vi "_readLabel_fromDatabase_wmg.vi"(0 "input_str_label":string="11S90Y9428Y050YW6154M1", 1 "SN keep":bool, 2 "date":timestamp, 3 "input_array_labelConfig":string[](array[string])=["年月日", "16", "16", "17", "17", "", "", "18", "18", "19", "21", "Y050YW(YMD)(S3)"]) -> (4 "show_str_yywwSd":string, 5 "show_str_yydddxxxx":string, 6 "show_int_Xn":i32, 7 "show_date":timestamp format="%<%X\n%x>T", 8 "show_str_snObeyFormat":string="LR5AN0021")   [LabVIEW 2011]
panel:
  in  "midVar_date_2":timestamp
  in  "midVar_date_1":timestamp
  # "周日是一周的第0天"
  # "1904050897/Z00A2R1543S500016\n0       5       10         17     22\nL99SF014-SD-H"
  # "8SSC10G59338L1DG5AN0004\nL01HE006-SD-R"
  # "1904050897/Z00A2R1543S500016\n0       5       10         17     22\nL99SF014-SD-H\n\n1543S5经本程序计算得到2015/10/23 296"
  # "这个输出接口估计用不到了"
  # "17 18"
  # "数组元素索引\n0  description\n1  yearStart\n2  yearEnd\n3  monthStart\n4  monthEnd\n5  weekStart\n6  weekEnd\n7  DayStart\n8  DayEnd\n9  snStart\n10 snEnd\n11  snFormat\n12  cableType\n13  preStaData\n14  significant\n15  noRetest"
  # "0  description"
  # "1  yearStart"
  # "8SSC10G59338L1DG5AN0004\n\nL01HE006-SD-R\n5AN经本程序计算得到2015/10/22 295\n\n8SSC10G59338L1DG5110004\nL01HE006-SD-R\n5AN经本程序计算得到2015/1/1 1"
  # "2  yearEnd"
  # "3  monthStart"
  # "4  monthEnd"
  # "5  weekStart"
  # "6  weekEnd"
  # "7  DayStart"
  # "8  DayEnd"
  # "9  snStart"
  # "10 snEnd"
  # "11  snFormat"
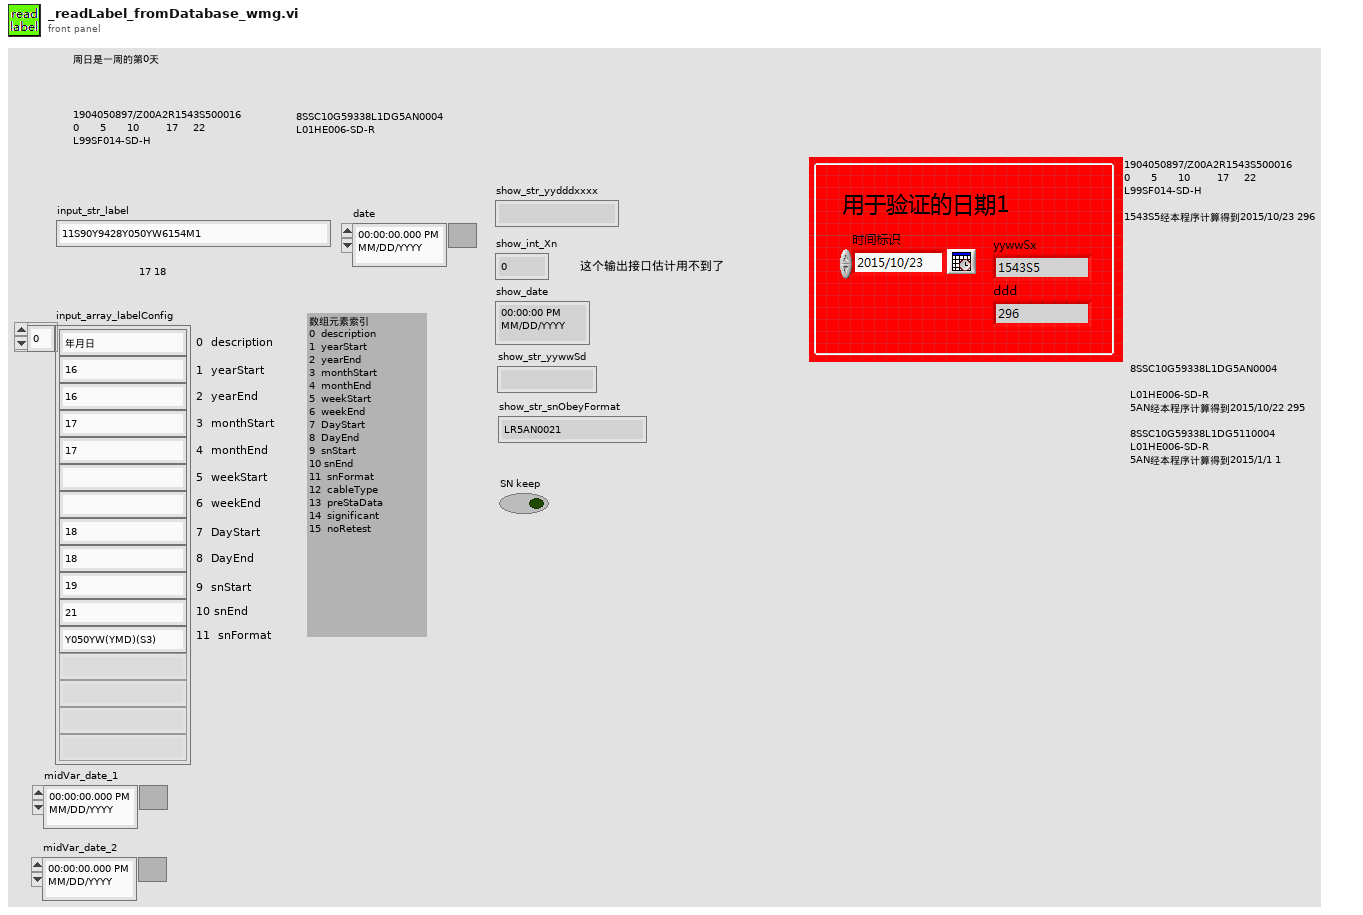
[diagram p1: front panel]
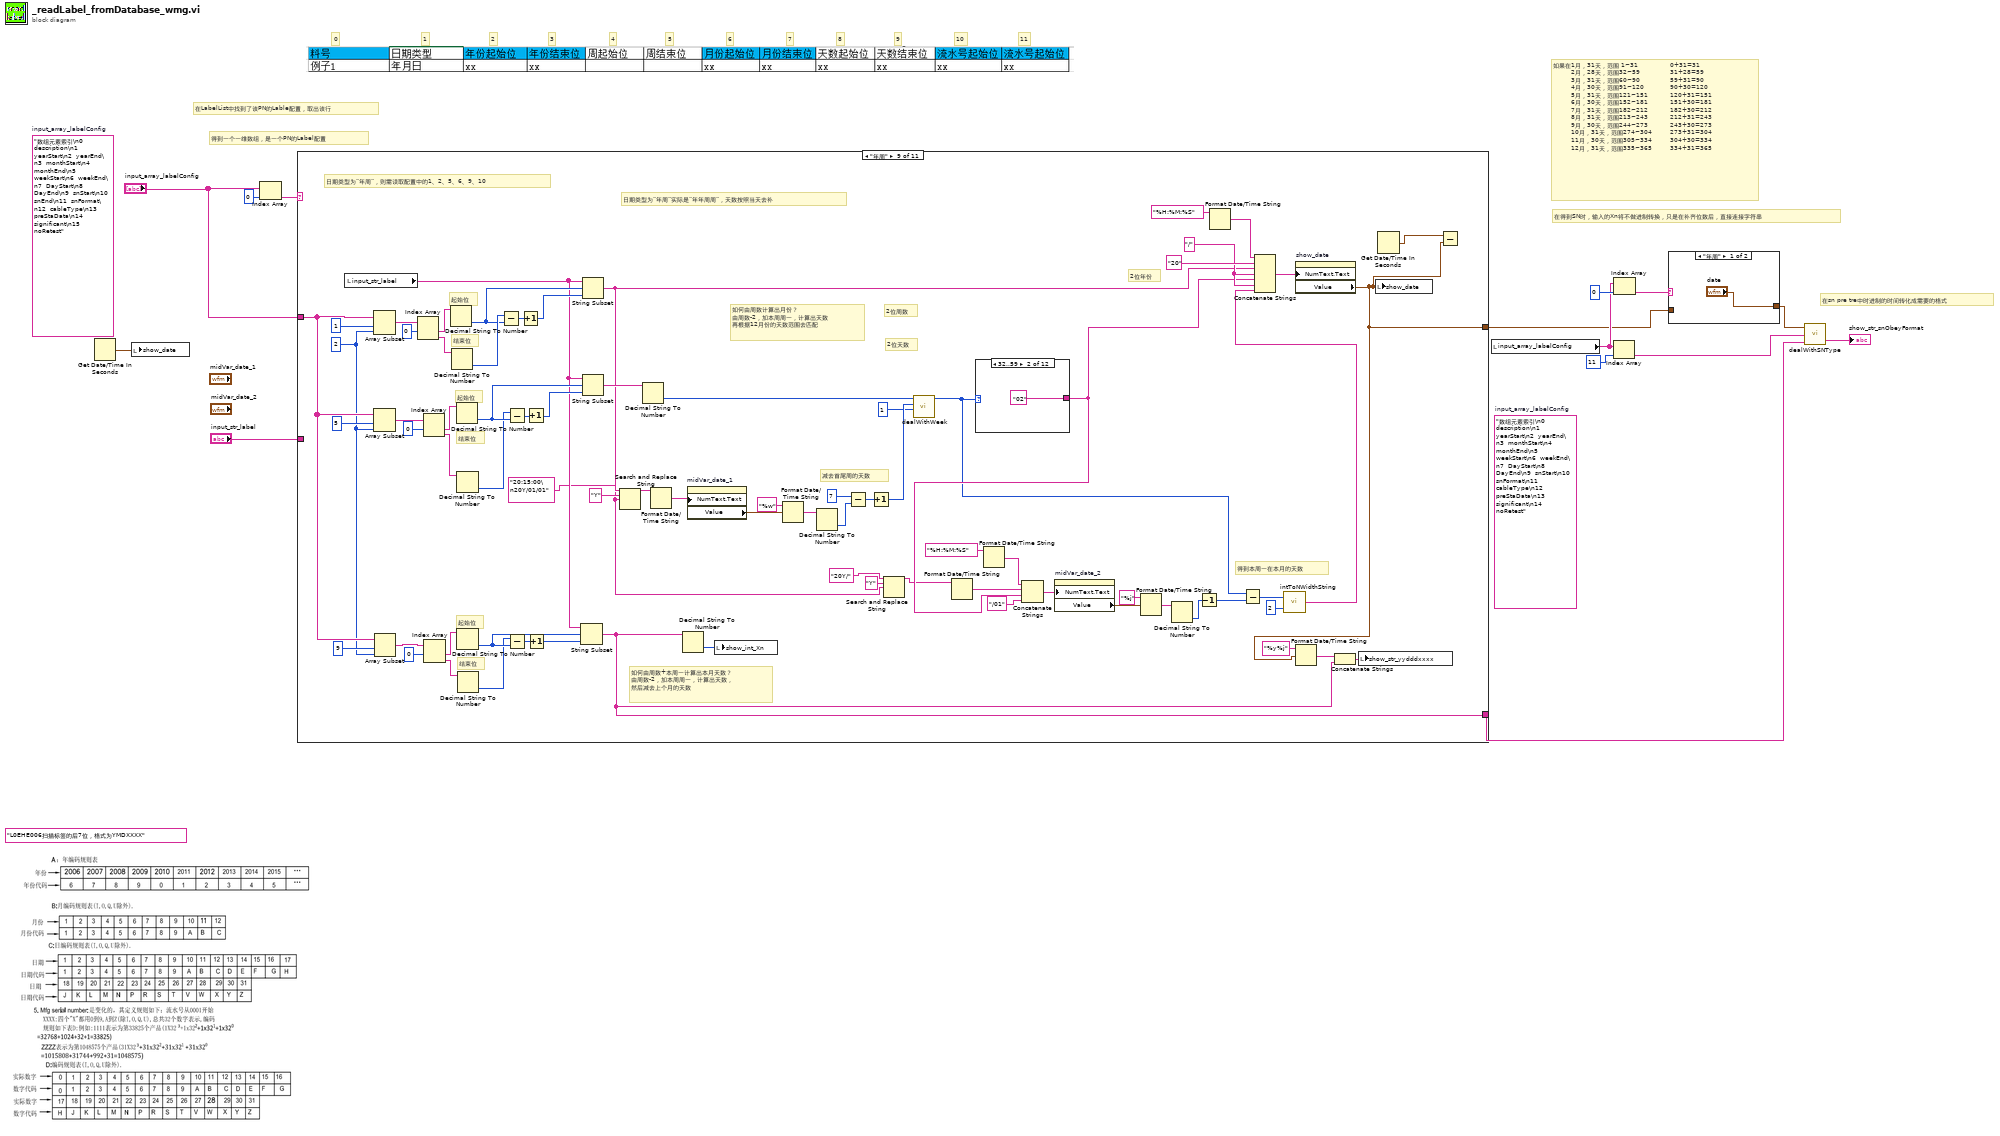
[diagram p0: block diagram]
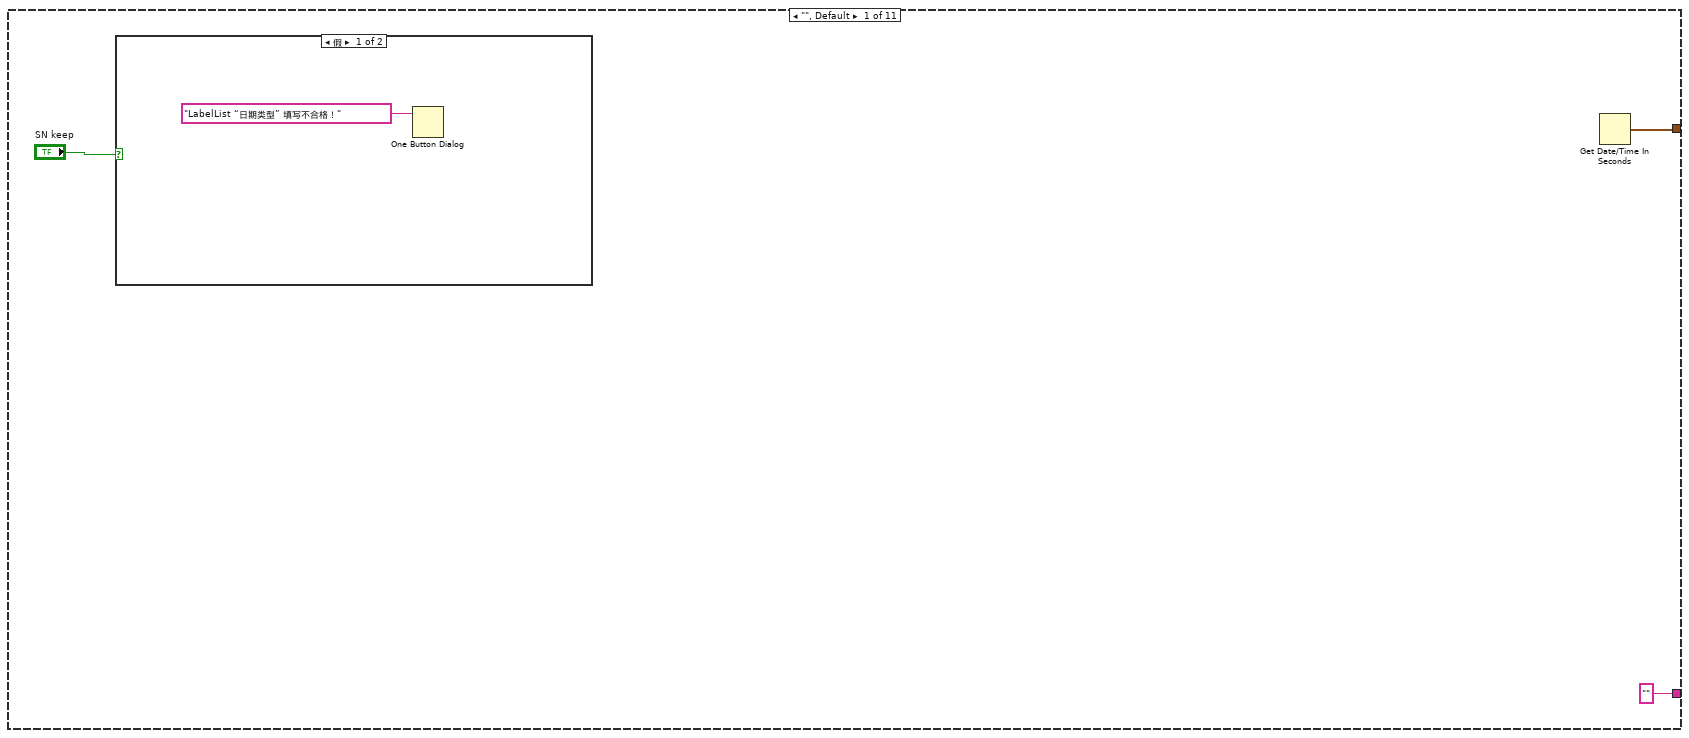
[diagram p3: hidden frame]
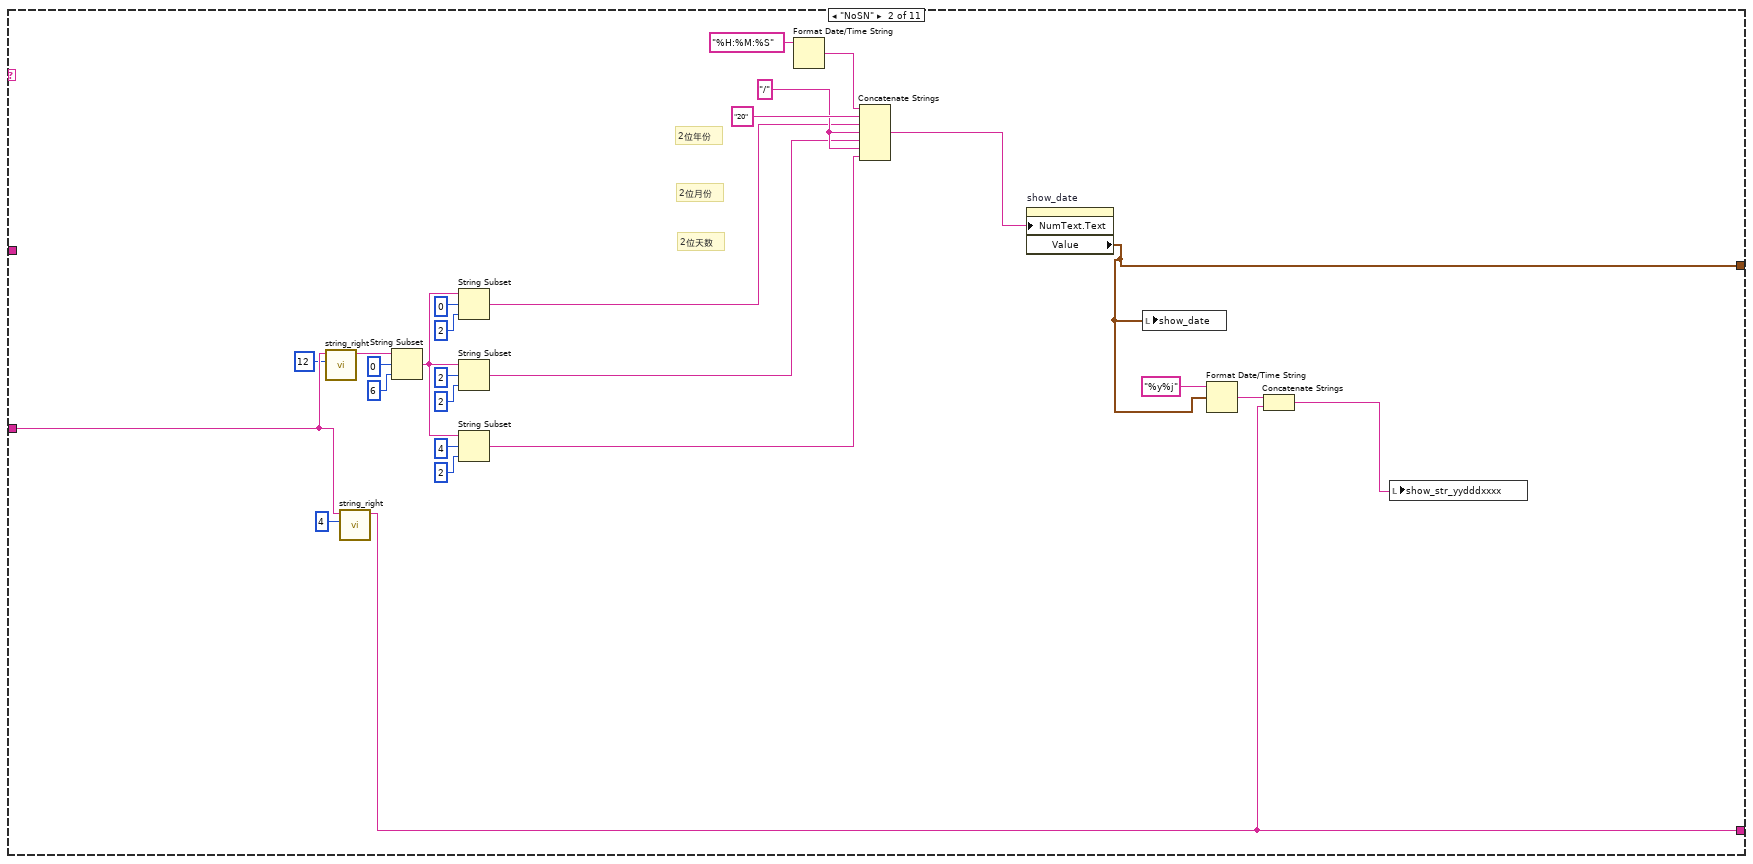
[diagram p5: hidden frame]
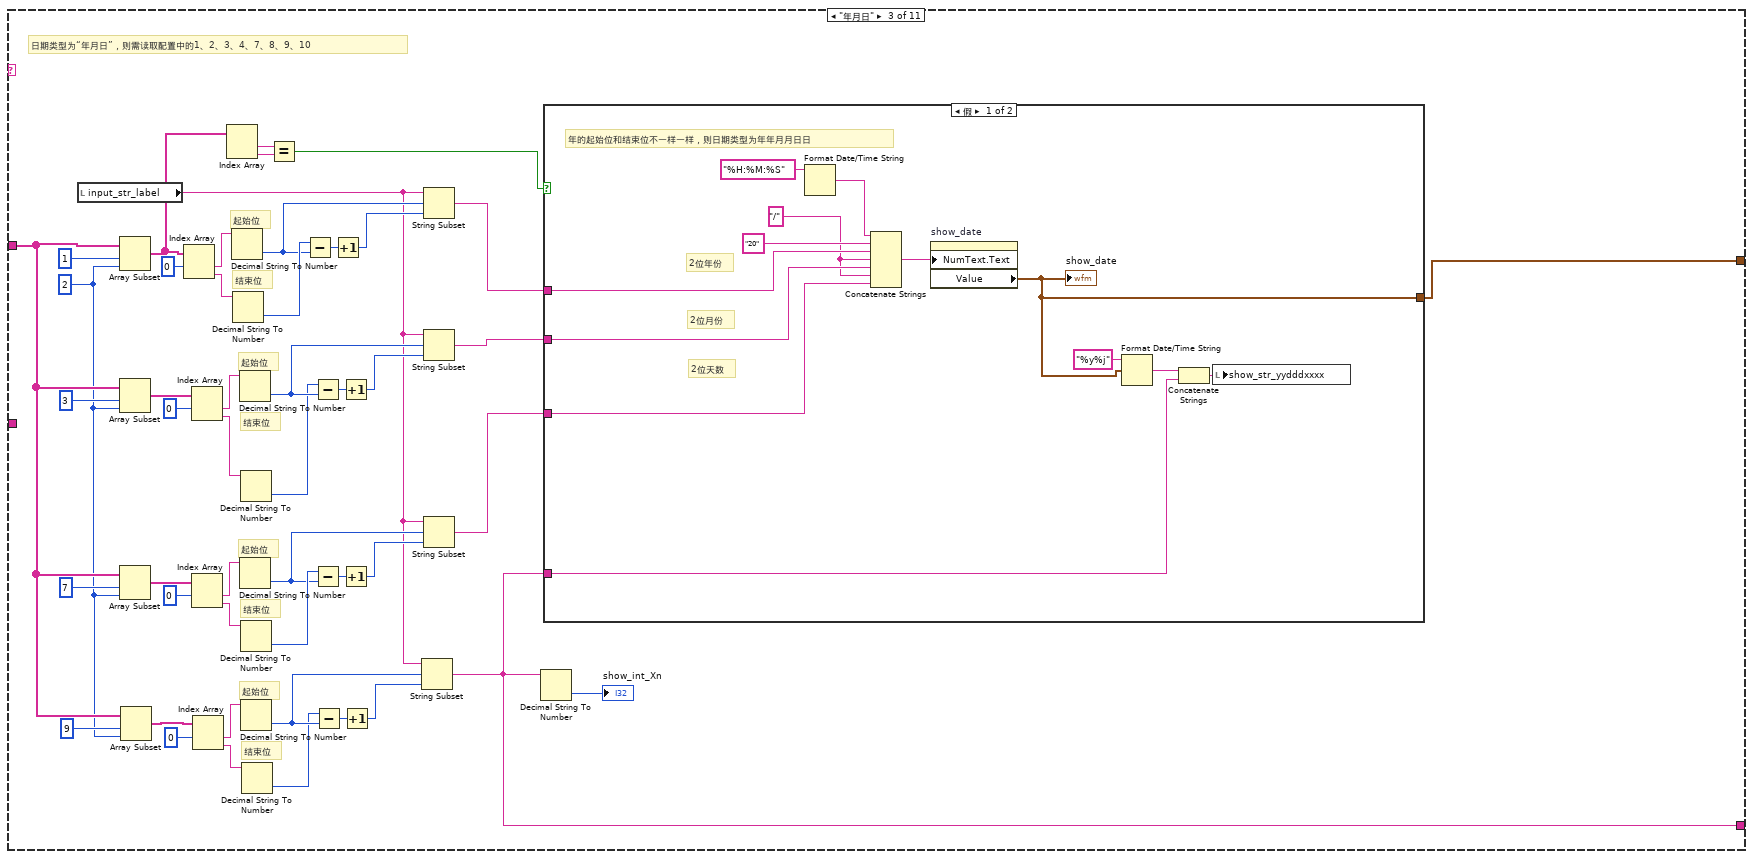
[diagram p6: hidden frame]
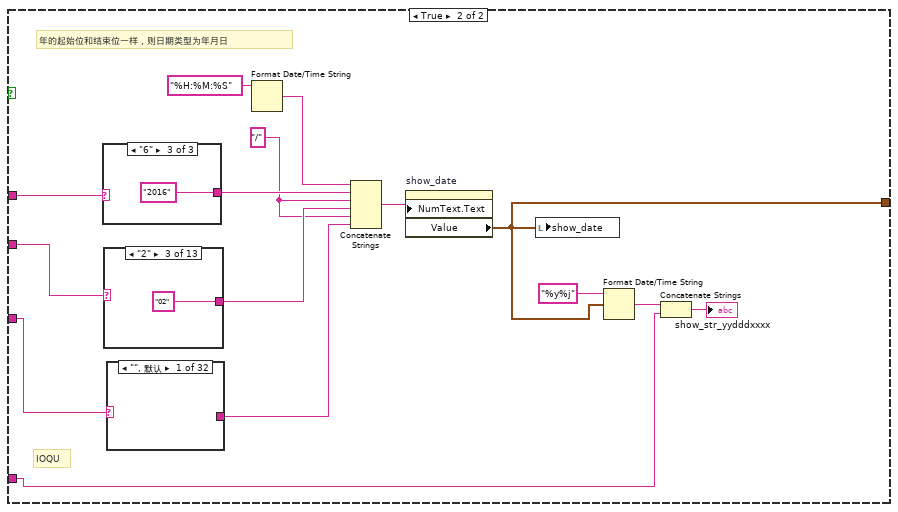
[diagram p7: hidden frame]
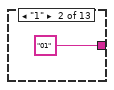
[diagram p9: hidden frame]
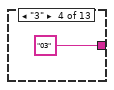
[diagram p10: hidden frame]
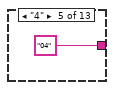
[diagram p11: hidden frame]
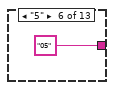
[diagram p12: hidden frame]
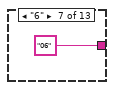
[diagram p13: hidden frame]
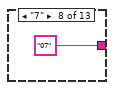
[diagram p14: hidden frame]
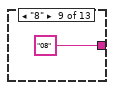
[diagram p15: hidden frame]
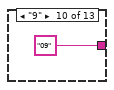
[diagram p16: hidden frame]
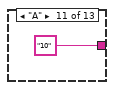
[diagram p17: hidden frame]
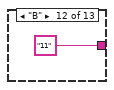
[diagram p18: hidden frame]
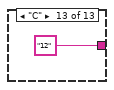
[diagram p19: hidden frame]
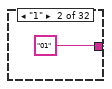
[diagram p20: hidden frame]
diagram:
  (unwired) "数组元素索引\n0  description\n1  yearStart\n2  yearEnd\n3  monthStart\n4  monthEnd\n5  weekStart\n6  weekEnd\n7  DayStart\n8  DayEnd\n9  snStart\n10  snFormat\n11  cableType\n12  preStaData\n13  significant\n14  noRetest"  # input_array_labelConfig
  (unwired) "数组元素索引\n0  description\n1  yearStart\n2  yearEnd\n3  monthStart\n4  monthEnd\n5  weekStart\n6  weekEnd\n7  DayStart\n8  DayEnd\n9  snStart\n10 snEnd\n11  snFormat\n12  cableType\n13  preStaData\n14  significant\n15  noRetest"  # input_array_labelConfig
  (unwired) "L0EHE006扫描标签的后7位，格式为YMDXXXX"
  # "在sn pre tre中时进制的时间转化成需要的格式"
  # "在得到SN时，输入的Xn将不做进制转换，只是在补齐位数后，直接连接字符串"
  # "得到一个一维数组，是一个PN的Label配置"
  # "在LabelList中找到了该PN的Lable配置，取出该行"
  # "如果在1月，31天，范围 1~31                0+31=31\n         2月，28天，范围32~59               31+28=59\n         3月，31天，范围60~90               59+31=90\n         4月，30天，范围91~120             90+30=120\n         5月，31天，范围121~151           120+31=151\n         6月，30天，范围152~181           151+30=181\n         7月，31天，范围182~212           182+30=212\n         8月，31天，范围213~243           212+31=243\n         9月，30天，范围244~273           243+30=273\n         10月，31天，范围274~304         273+31=304\n         11月，30天，范围305~334         304+30=334\n         12月，31天，范围335~365         334+31=365"
  # "11"
  # "10"
  # "9"
  # "8"
  # "7"
  # "6"
  # "5"
  # "4"
  # "3"
  # "2"
  # "1"
  # "0"
  n1 = Get Date/Time In Seconds() -> (seconds since 1Jan1904=w14:timestamp)
  n2 = local write "show_date"(w14) -> ()
  n3 = Index Array(array="input_array_labelConfig", index=0 ("索引")) -> (element=w12:string)
  n4 = case shown="\"年周\"" w12 {
    tunnel: "input_array_labelConfig" -> [_ _ w89 w210 w338 w465 w546 w600 w756 w792 w882]
    tunnel: [w17 w19 w46 w168 w297 w424 w542 w559 w684 w779 w891] -> w3
    tunnel: ["" ("input_str_label") w21 w45 w167 w288 w417 w544 w556 w699 w778 w890] -> w8
    tunnel: "input_str_label" -> [_ w43 _ _ _ _ w543 _ _ _ _]
    frame "", Default {
      n5 = case shown="假" "SN keep" {
        frame False {
          n6 = One Button Dialog(message="LabelList “日期类型” 填写不合格！") -> ()  [unwired: 1 in, 1 out]
        }
        frame True {
        }
      }
      n7 = Get Date/Time In Seconds() -> (seconds since 1Jan1904=w17:timestamp)
    }
    frame "NoSN" {
      w37 = "/"
      # "2位天数"
      # "2位月份"
      # "2位年份"
      n8 = call "string_right.vi"("length"=12, "string"=w43) -> ("to"=w41:string)  [unwired: 9 in]
      n9 = call "string_right.vi"("length"=4, "string"=w43) -> ("to"=w21:string)  [unwired: 9 in]
      n10 = String Subset(string=w41, offset (0)=0 ("偏移量(0)"), length (rest)=6 ("长度（剩余）")) -> (substring=w26:string)
      n11 = String Subset(string=w26, offset (0)=0 ("偏移量(0)"), length (rest)=2 ("长度（剩余）")) -> (substring=w32:string)
      n12 = String Subset(string=w26, offset (0)=2 ("偏移量(0)"), length (rest)=2 ("长度（剩余）")) -> (substring=w29:string)
      n13 = String Subset(string=w26, offset (0)=4 ("偏移量(0)"), length (rest)=2 ("长度（剩余）")) -> (substring=w25:string)
      n14 = Format Date/Time String(time format string (%c)="%H:%M:%S" ("时间格式字符串(%c)")) -> (date/time string=w35:string)  [unwired: 2 in]
      n15 = Concatenate Strings(w35, "20", w32, w37, w29, w37, w25) -> (w22:string)
      n16 = property on="show_date" class="AbsTime (严格)"("NumText.Text"=w22) -> ("Value"=w19:timestamp)  [unwired: 2 in, 2 out]
      n17 = local write "show_date"(w19) -> ()
      n18 = Format Date/Time String(time format string (%c)="%y%j" ("时间格式字符串(%c)"), seconds (now)=w19) -> (date/time string=w23:string)  [unwired: 1 in]
      n19 = Concatenate Strings(w23, w21) -> (w20:string)
      n20 = local write "show_str_yydddxxxx"(w20) -> ()
    }
    frame "年月日" {
      w47 = 2 ("索引")
      # "结束位"
      # "起始位"
      # "结束位"
      # "起始位"
      # "结束位"
      # "起始位"
      # "结束位"
      # "起始位"
      # "日期类型为“年月日”，则需读取配置中的1、2、3、4、7、8、9、10"
      n21 = local read "input_str_label"() -> (w50:string)
      n22 = Array Subset(array=w89, index=1 ("索引"), length=w47) -> (w84:string[])
      n23 = Array Subset(array=w89, index=3 ("索引"), length=w47) -> (w71:string[])
      n24 = Array Subset(array=w89, index=7 ("索引"), length=w47) -> (w63:string[])
      n25 = Array Subset(array=w89, index=9 ("索引"), length=w47) -> (w51:string[])
      n26 = Index Array(array=w84, index #1=0 ("索引")) -> (element #1=w83:string, element #2=w82:string)  [unwired: 1 in]
      n27 = Index Array(array=w71, index #1=0 ("索引")) -> (element #1=w73:string, element #2=w74:string)  [unwired: 1 in]
      n28 = Index Array(array=w63, index #1=0 ("索引")) -> (element #1=w64:string, element #2=w68:string)  [unwired: 1 in]
      n29 = Index Array(array=w51, index #1=0 ("索引")) -> (element #1=w57:string, element #2=w53:string)  [unwired: 1 in]
      n30 = Index Array(array=w84) -> (element #1=w88:string, element #2=w87:string)  [unwired: 2 in]
      n31 = Decimal String To Number(string=w83) -> (number=w80:i32)  [unwired: 2 in, 1 out]
      n32 = Decimal String To Number(string=w82) -> (number=w81:i32)  [unwired: 2 in, 1 out]
      n33 = Decimal String To Number(string=w73) -> (number=w76:i32)  [unwired: 2 in, 1 out]
      n34 = Decimal String To Number(string=w64) -> (number=w66:i32)  [unwired: 2 in, 1 out]
      n35 = Decimal String To Number(string=w74) -> (number=w75:i32)  [unwired: 2 in, 1 out]
      n36 = Decimal String To Number(string=w68) -> (number=w67:i32)  [unwired: 2 in, 1 out]
      n37 = Decimal String To Number(string=w57) -> (number=w55:i32)  [unwired: 2 in, 1 out]
      n38 = Decimal String To Number(string=w53) -> (number=w54:i32)  [unwired: 2 in, 1 out]
      n39 = Equal?(x=w88, y=w87) -> (x = y?=w86:bool)
      n40 = Subtract(x=w81, y=w80) -> (x-y=w85:i32)
      n41 = Subtract(x=w75, y=w76) -> (x-y=w72:i32)
      n42 = Subtract(x=w67, y=w66) -> (x-y=w69:i32)
      n43 = Subtract(x=w54, y=w55) -> (x-y=w52:i32)
      n44 = Increment(x=w85) -> (x+1=w79:i32)
      n45 = Increment(x=w72) -> (x+1=w77:i32)
      n46 = Increment(x=w69) -> (x+1=w65:i32)
      n47 = Increment(x=w52) -> (x+1=w56:i32)
      n48 = String Subset(string=w50, offset (0)=w55, length (rest)=w56) -> (substring=w45:string)
      n49 = String Subset(string=w50, offset (0)=w80, length (rest)=w79) -> (substring=w78:string)
      n50 = String Subset(string=w50, offset (0)=w76, length (rest)=w77) -> (substring=w70:string)
      n51 = String Subset(string=w50, offset (0)=w66, length (rest)=w65) -> (substring=w59:string)
      n52 = Decimal String To Number(string=w45) -> (number=→"show_int_Xn":i32)  [unwired: 2 in, 1 out]
      n53 = case shown="假" w86 {
        tunnel: w78 -> [w104 w120]
        tunnel: w70 -> [w103 w118]
        tunnel: w59 -> [w101 w119]
        tunnel: w45 -> [w93 w106]
        tunnel: [w94 w107] -> w46
        frame False {
          w102 = "/"
          # "年的起始位和结束位不一样一样，则日期类型为年年月月日日"
          # "2位天数"
          # "2位月份"
          # "2位年份"
          n54 = Format Date/Time String(time format string (%c)="%H:%M:%S" ("时间格式字符串(%c)")) -> (date/time string=w99:string)  [unwired: 2 in]
          n55 = Concatenate Strings(w99, "20", w104, w102, w103, w102, w101) -> (w98:string)
          n56 = property on="show_date" class="AbsTime (严格)"("NumText.Text"=w98) -> ("Value"=w94:timestamp)  [unwired: 2 in, 2 out]
          "show_date" <- w94
          n57 = Format Date/Time String(time format string (%c)="%y%j" ("时间格式字符串(%c)"), seconds (now)=w94) -> (date/time string=w96:string)  [unwired: 1 in]
          n58 = Concatenate Strings(w96, w93) -> (w97:string)
          n59 = local write "show_str_yydddxxxx"(w97) -> ()
        }
        frame True {
          w113 = "/"
          # "IOQU"
          # "年的起始位和结束位一样，则日期类型为年月日"
          n60 = case shown="\"6\"" w120 {
            tunnel: [_ "2015" "2016"] -> w117
            frame Default {
            }
            frame "5" {
            }
            frame "6" {
            }
          }
          n61 = case shown="\"2\"" w118 {
            tunnel: [_ "01" "02" "03" "04" "05" "06" "07" "08" "09" "10" "11" "12"] -> w114
            frame "", Default {
            }
            frame "1" {
            }
            frame "2" {
            }
            frame "3" {
            }
            frame "4" {
            }
            frame "5" {
            }
            frame "6" {
            }
            frame "7" {
            }
            frame "8" {
            }
            frame "9" {
            }
            frame "A" {
            }
            frame "B" {
            }
            frame "C" {
            }
          }
          n62 = case shown="\"\", 默认" w119 {
            tunnel: [_ "01" "02" "03" "04" "05" "06" "07" "08" "09" "10" "11" "12" "13" "14" "15" "16" "17" "18" "19" "20" "21" "22" "23" "24" "25" "26" "27" "28" "29" "30" "31"] -> w112
            frame "", Default {
            }
            frame "1" {
            }
            frame "2" {
            }
            frame "3" {
            }
            frame "4" {
            }
            frame "5" {
            }
            frame "6" {
            }
            frame "7" {
            }
            frame "8" {
            }
            frame "9" {
            }
            frame "A" {
            }
            frame "B" {
            }
            frame "C" {
            }
            frame "D" {
            }
            frame "E" {
            }
            frame "F" {
            }
            frame "G" {
            }
            frame "H" {
            }
            frame "J" {
            }
            frame "K" {
            }
            frame "L" {
            }
            frame "M" {
            }
            frame "N" {
            }
            frame "P" {
            }
            frame "R" {
            }
            frame "S" {
            }
            frame "T" {
            }
            frame "V" {
            }
            frame "W" {
            }
            frame "X" {
            }
            frame "Y" {
            }
            frame "Z" {
            }
          }
          n63 = Format Date/Time String(time format string (%c)="%H:%M:%S" ("时间格式字符串(%c)")) -> (date/time string=w115:string)  [unwired: 2 in]
          n64 = Concatenate Strings(w115, w117, w113, w114, w113, w112) -> (w111:string)
          n65 = property on="show_date" class="AbsTime (严格)"("NumText.Text"=w111) -> ("Value"=w107:timestamp)  [unwired: 2 in, 2 out]
          n66 = local write "show_date"(w107) -> ()
          n67 = Format Date/Time String(time format string (%c)="%y%j" ("时间格式字符串(%c)"), seconds (now)=w107) -> (date/time string=w109:string)  [unwired: 1 in]
          n68 = Concatenate Strings(w109, w106) -> (→"show_str_yydddxxxx":string)
        }
      }
    }
    frame "年月日4" {
      w169 = 2 ("索引")
      # "结束位"
      # "起始位"
      # "结束位"
      # "起始位"
      # "结束位"
      # "起始位"
      # "结束位"
      # "起始位"
      # "日期类型为“年月日”，则需读取配置中的1、2、3、4、7、8、9、10"
      n69 = local read "input_str_label"() -> (w171:string)
      n70 = Array Subset(array=w210, index=1 ("索引"), length=w169) -> (w205:string[])
      n71 = Array Subset(array=w210, index=3 ("索引"), length=w169) -> (w192:string[])
      n72 = Array Subset(array=w210, index=7 ("索引"), length=w169) -> (w184:string[])
      n73 = Array Subset(array=w210, index=9 ("索引"), length=w169) -> (w172:string[])
      n74 = Index Array(array=w205, index #1=0 ("索引")) -> (element #1=w204:string, element #2=w203:string)  [unwired: 1 in]
      n75 = Index Array(array=w192, index #1=0 ("索引")) -> (element #1=w194:string, element #2=w195:string)  [unwired: 1 in]
      n76 = Index Array(array=w184, index #1=0 ("索引")) -> (element #1=w185:string, element #2=w189:string)  [unwired: 1 in]
      n77 = Index Array(array=w172, index #1=0 ("索引")) -> (element #1=w178:string, element #2=w174:string)  [unwired: 1 in]
      n78 = Index Array(array=w205) -> (element #1=w209:string, element #2=w208:string)  [unwired: 2 in]
      n79 = Decimal String To Number(string=w204) -> (number=w201:i32)  [unwired: 2 in, 1 out]
      n80 = Decimal String To Number(string=w203) -> (number=w202:i32)  [unwired: 2 in, 1 out]
      n81 = Decimal String To Number(string=w194) -> (number=w197:i32)  [unwired: 2 in, 1 out]
      n82 = Decimal String To Number(string=w185) -> (number=w187:i32)  [unwired: 2 in, 1 out]
      n83 = Decimal String To Number(string=w195) -> (number=w196:i32)  [unwired: 2 in, 1 out]
      n84 = Decimal String To Number(string=w189) -> (number=w188:i32)  [unwired: 2 in, 1 out]
      n85 = Decimal String To Number(string=w178) -> (number=w176:i32)  [unwired: 2 in, 1 out]
      n86 = Decimal String To Number(string=w174) -> (number=w175:i32)  [unwired: 2 in, 1 out]
      n87 = Equal?(x=w209, y=w208) -> (x = y?=w207:bool)
      n88 = Subtract(x=w202, y=w201) -> (x-y=w206:i32)
      n89 = Subtract(x=w196, y=w197) -> (x-y=w193:i32)
      n90 = Subtract(x=w188, y=w187) -> (x-y=w190:i32)
      n91 = Subtract(x=w175, y=w176) -> (x-y=w173:i32)
      n92 = Increment(x=w206) -> (x+1=w200:i32)
      n93 = Increment(x=w193) -> (x+1=w198:i32)
      n94 = Increment(x=w190) -> (x+1=w186:i32)
      n95 = Increment(x=w173) -> (x+1=w177:i32)
      n96 = String Subset(string=w171, offset (0)=w176, length (rest)=w177) -> (substring=w167:string)
      n97 = String Subset(string=w171, offset (0)=w201, length (rest)=w200) -> (substring=w199:string)
      n98 = String Subset(string=w171, offset (0)=w197, length (rest)=w198) -> (substring=w191:string)
      n99 = String Subset(string=w171, offset (0)=w187, length (rest)=w186) -> (substring=w180:string)
      n100 = Decimal String To Number(string=w167) -> (number=w166:i32)  [unwired: 2 in, 1 out]
      n101 = case shown="真" w207 {
        tunnel: w199 -> [w225 w241]
        tunnel: w191 -> [w224 w239]
        tunnel: w180 -> [w222 w240]
        tunnel: w167 -> [w216 w229]
        tunnel: [w215 w228] -> w168
        frame False {
          w223 = "/"
          # "年的起始位和结束位不一样一样，则日期类型为年年月月日日"
          # "2位天数"
          # "2位月份"
          # "2位年份"
          n102 = Format Date/Time String(time format string (%c)="%H:%M:%S" ("时间格式字符串(%c)")) -> (date/time string=w220:string)  [unwired: 2 in]
          n103 = Concatenate Strings(w220, "20", w225, w223, w224, w223, w222) -> (w219:string)
          n104 = property on="show_date" class="AbsTime (严格)"("NumText.Text"=w219) -> ("Value"=w215:timestamp)  [unwired: 2 in, 2 out]
          n105 = local write "show_date"(w215) -> ()
          n106 = Format Date/Time String(time format string (%c)="%y%j" ("时间格式字符串(%c)"), seconds (now)=w215) -> (date/time string=w218:string)  [unwired: 1 in]
          n107 = Concatenate Strings(w218, w216) -> (w214:string)
          n108 = local write "show_str_yydddxxxx"(w214) -> ()
        }
        frame True {
          w234 = "/"
          # "IOQ"
          # "年的起始位和结束位一样，则日期类型为年月日"
          n109 = case shown="\"6\"" w241 {
            tunnel: [_ "2015" "2016"] -> w238
            frame Default {
            }
            frame "5" {
            }
            frame "6" {
            }
          }
          n110 = case shown="\"2\"" w239 {
            tunnel: [_ "01" "02" "03" "04" "05" "06" "07" "08" "09" "10" "11" "12"] -> w235
            frame "", Default {
            }
            frame "1" {
            }
            frame "2" {
            }
            frame "3" {
            }
            frame "4" {
            }
            frame "5" {
            }
            frame "6" {
            }
            frame "7" {
            }
            frame "8" {
            }
            frame "9" {
            }
            frame "A" {
            }
            frame "B" {
            }
            frame "C" {
            }
          }
          n111 = case shown="\"Z\"" w240 {
            tunnel: [_ "01" "02" "03" "04" "05" "06" "07" "08" "09" "10" "11" "12" "13" "14" "15" "16" "17" "18" "19" "20" "21" "22" "23" "24" "25" "26" "27" "28" "29" "30" "31" "32"] -> w233
            frame "", Default {
            }
            frame "1" {
            }
            frame "2" {
            }
            frame "3" {
            }
            frame "4" {
            }
            frame "5" {
            }
            frame "6" {
            }
            frame "7" {
            }
            frame "8" {
            }
            frame "9" {
            }
            frame "A" {
            }
            frame "B" {
            }
            frame "C" {
            }
            frame "D" {
            }
            frame "E" {
            }
            frame "F" {
            }
            frame "G" {
            }
            frame "H" {
            }
            frame "J" {
            }
            frame "K" {
            }
            frame "L" {
            }
            frame "M" {
            }
            frame "N" {
            }
            frame "P" {
            }
            frame "R" {
            }
            frame "S" {
            }
            frame "T" {
            }
            frame "U" {
            }
            frame "V" {
            }
            frame "W" {
            }
            frame "X" {
            }
            frame "Y" {
            }
            frame "Z" {
            }
          }
          n112 = Format Date/Time String(time format string (%c)="%H:%M:%S" ("时间格式字符串(%c)")) -> (date/time string=w236:string)  [unwired: 2 in]
          n113 = Concatenate Strings(w236, w238, w234, w235, w234, w233) -> (w232:string)
          n114 = property on="show_date" class="AbsTime (严格)"("NumText.Text"=w232) -> ("Value"=w228:timestamp)  [unwired: 2 in, 2 out]
          n115 = local write "show_date"(w228) -> ()
          n116 = Format Date/Time String(time format string (%c)="%y%j" ("时间格式字符串(%c)"), seconds (now)=w228) -> (date/time string=w230:string)  [unwired: 1 in]
          n117 = Concatenate Strings(w230, w229) -> (w227:string)
          n118 = local write "show_str_yydddxxxx"(w227) -> ()
        }
      }
      n119 = local write "show_int_Xn"(w166) -> ()
    }
    frame "年月日2" {
      w298 = 2 ("索引")
      # "结束位"
      # "起始位"
      # "结束位"
      # "起始位"
      # "结束位"
      # "起始位"
      # "结束位"
      # "起始位"
      # "日期类型为“年月日”，则需读取配置中的1、2、3、4、7、8、9、10"
      n120 = local read "input_str_label"() -> (w300:string)
      n121 = Array Subset(array=w338, index=1 ("索引"), length=w298) -> (w333:string[])
      n122 = Array Subset(array=w338, index=3 ("索引"), length=w298) -> (w320:string[])
      n123 = Array Subset(array=w338, index=7 ("索引"), length=w298) -> (w312:string[])
      n124 = Array Subset(array=w338, index=9 ("索引"), length=w298) -> (w301:string[])
      n125 = Index Array(array=w333, index #1=0 ("索引")) -> (element #1=w332:string, element #2=w331:string)  [unwired: 1 in]
      n126 = Index Array(array=w320, index #1=0 ("索引")) -> (element #1=w322:string, element #2=w323:string)  [unwired: 1 in]
      n127 = Index Array(array=w312, index #1=0 ("索引")) -> (element #1=w313:string, element #2=w317:string)  [unwired: 1 in]
      n128 = Index Array(array=w301, index #1=0 ("索引")) -> (element #1=w306:string, element #2=w303:string)  [unwired: 1 in]
      n129 = Index Array(array=w333) -> (element #1=w337:string, element #2=w336:string)  [unwired: 2 in]
      n130 = Decimal String To Number(string=w332) -> (number=w329:i32)  [unwired: 2 in, 1 out]
      n131 = Decimal String To Number(string=w331) -> (number=w330:i32)  [unwired: 2 in, 1 out]
      n132 = Decimal String To Number(string=w322) -> (number=w325:i32)  [unwired: 2 in, 1 out]
      n133 = Decimal String To Number(string=w313) -> (number=w315:i32)  [unwired: 2 in, 1 out]
      n134 = Decimal String To Number(string=w323) -> (number=w324:i32)  [unwired: 2 in, 1 out]
      n135 = Decimal String To Number(string=w317) -> (number=w316:i32)  [unwired: 2 in, 1 out]
      n136 = Decimal String To Number(string=w306) -> (number=w305:i32)  [unwired: 2 in, 1 out]
      n137 = Decimal String To Number(string=w303) -> (number=w304:i32)  [unwired: 2 in, 1 out]
      n138 = Equal?(x=w337, y=w336) -> (x = y?=w335:bool)
      n139 = Subtract(x=w330, y=w329) -> (x-y=w334:i32)
      n140 = Subtract(x=w324, y=w325) -> (x-y=w321:i32)
      n141 = Subtract(x=w316, y=w315) -> (x-y=w318:i32)
      n142 = Subtract(x=w304, y=w305) -> (x-y=w302:i32)
      n143 = Increment(x=w334) -> (x+1=w328:i32)
      n144 = Increment(x=w321) -> (x+1=w326:i32)
      n145 = Increment(x=w318) -> (x+1=w314:i32)
      n146 = Increment(x=w302) -> (x+1=w293:i32)
      n147 = String Subset(string=w300, offset (0)=w305, length (rest)=w293) -> (substring=w295:string)
      n148 = String Subset(string=w300, offset (0)=w329, length (rest)=w328) -> (substring=w327:string)
      n149 = String Subset(string=w300, offset (0)=w325, length (rest)=w326) -> (substring=w319:string)
      n150 = String Subset(string=w300, offset (0)=w315, length (rest)=w314) -> (substring=w308:string)
      n151 = Decimal String To Number(string=w295) -> (number=w296:i32)  [unwired: 2 in, 1 out]
      n152 = case shown="真" w335 {
        tunnel: w327 -> [w353 w369]
        tunnel: w319 -> [w352 w367]
        tunnel: w308 -> [w350 w368]
        tunnel: w295 -> [w344 w356]
        tunnel: [w343 w357] -> w297
        frame False {
          w351 = "/"
          # "年的起始位和结束位不一样一样，则日期类型为年年月月日日"
          # "2位天数"
          # "2位月份"
          # "2位年份"
          n153 = Format Date/Time String(time format string (%c)="%H:%M:%S" ("时间格式字符串(%c)")) -> (date/time string=w348:string)  [unwired: 2 in]
          n154 = Concatenate Strings(w348, "20", w353, w351, w352, w351, w350) -> (w347:string)
          n155 = property on="show_date" class="AbsTime (严格)"("NumText.Text"=w347) -> ("Value"=w343:timestamp)  [unwired: 2 in, 2 out]
          n156 = local write "show_date"(w343) -> ()
          n157 = Format Date/Time String(time format string (%c)="%y%j" ("时间格式字符串(%c)"), seconds (now)=w343) -> (date/time string=w346:string)  [unwired: 1 in]
          n158 = Concatenate Strings(w346, w344) -> (w342:string)
          n159 = local write "show_str_yydddxxxx"(w342) -> ()
        }
        frame True {
          w362 = "/"
          # "IOQU"
          # "年的起始位和结束位一样，则日期类型为年月日"
          n160 = case shown="\"6\"" w369 {
            tunnel: [_ "2015" "2016"] -> w366
            frame Default {
            }
            frame "5" {
            }
            frame "6" {
            }
          }
          n161 = case shown="\"C\"" w367 {
            tunnel: [_ "01" "02" "03" "04" "05" "06" "07" "08" "09" "10" "11" "12"] -> w363
            frame "", Default {
            }
            frame "1" {
            }
            frame "2" {
            }
            frame "3" {
            }
            frame "4" {
            }
            frame "5" {
            }
            frame "6" {
            }
            frame "7" {
            }
            frame "8" {
            }
            frame "9" {
            }
            frame "A" {
            }
            frame "B" {
            }
            frame "C" {
            }
          }
          n162 = case shown="\"V\"" w368 {
            tunnel: [_ "01" "02" "03" "04" "05" "06" "07" "08" "09" "10" "11" "12" "13" "14" "15" "16" "17" "18" "19" "20" "21" "22" "23" "24" "25" "26" "27" "28" "29" "30" "31"] -> w361
            frame "", Default {
            }
            frame "1" {
            }
            frame "2" {
            }
            frame "3" {
            }
            frame "4" {
            }
            frame "5" {
            }
            frame "6" {
            }
            frame "7" {
            }
            frame "8" {
            }
            frame "9" {
            }
            frame "A" {
            }
            frame "B" {
            }
            frame "C" {
            }
            frame "D" {
            }
            frame "E" {
            }
            frame "F" {
            }
            frame "G" {
            }
            frame "H" {
            }
            frame "I" {
            }
            frame "J" {
            }
            frame "K" {
            }
            frame "L" {
            }
            frame "M" {
            }
            frame "N" {
            }
            frame "O" {
            }
            frame "P" {
            }
            frame "Q" {
            }
            frame "R" {
            }
            frame "S" {
            }
            frame "T" {
            }
            frame "U" {
            }
            frame "V" {
            }
          }
          n163 = Format Date/Time String(time format string (%c)="%H:%M:%S" ("时间格式字符串(%c)")) -> (date/time string=w364:string)  [unwired: 2 in]
          n164 = Concatenate Strings(w364, w366, w362, w363, w362, w361) -> (w360:string)
          n165 = property on="show_date" class="AbsTime (严格)"("NumText.Text"=w360) -> ("Value"=w357:timestamp)  [unwired: 2 in, 2 out]
          n166 = local write "show_date"(w357) -> ()
          n167 = Format Date/Time String(time format string (%c)="%y%j" ("时间格式字符串(%c)"), seconds (now)=w357) -> (date/time string=w358:string)  [unwired: 1 in]
          n168 = Concatenate Strings(w358, w356) -> (w355:string)
          n169 = local write "show_str_yydddxxxx"(w355) -> ()
        }
      }
      n170 = local write "show_int_Xn"(w296) -> ()
      n171 = call "25StrToDecStr_dell.vi"("input_str_hex"=w295) -> ("数值"=w294:i32)
      n172 = Number To Decimal String(number=w294, width (-)=w293) -> (decimal integer string=w292:string)
      n173 = Search and Replace String(replace all?=TRUE ("替换全部？(F)"), input string=w292, search string=" " ("搜索字符串"), replace string="0" ("替换字符串(\"\")")) -> (result string=w288:string)  [unwired: 4 in, 3 out]
    }
    frame "年月日5" {
      w425 = 2 ("索引")
      # "结束位"
      # "起始位"
      # "结束位"
      # "起始位"
      # "结束位"
      # "起始位"
      # "结束位"
      # "起始位"
      # "日期类型为“年月日”，则需读取配置中的1、2、3、4、7、8、9、10"
      n174 = local read "input_str_label"() -> (w427:string)
      n175 = Array Subset(array=w465, index=1 ("索引"), length=w425) -> (w460:string[])
      n176 = Array Subset(array=w465, index=3 ("索引"), length=w425) -> (w447:string[])
      n177 = Array Subset(array=w465, index=7 ("索引"), length=w425) -> (w439:string[])
      n178 = Array Subset(array=w465, index=9 ("索引"), length=w425) -> (w428:string[])
      n179 = Index Array(array=w460, index #1=0 ("索引")) -> (element #1=w459:string, element #2=w458:string)  [unwired: 1 in]
      n180 = Index Array(array=w447, index #1=0 ("索引")) -> (element #1=w449:string, element #2=w450:string)  [unwired: 1 in]
      n181 = Index Array(array=w439, index #1=0 ("索引")) -> (element #1=w440:string, element #2=w444:string)  [unwired: 1 in]
      n182 = Index Array(array=w428, index #1=0 ("索引")) -> (element #1=w433:string, element #2=w430:string)  [unwired: 1 in]
      n183 = Index Array(array=w460) -> (element #1=w464:string, element #2=w463:string)  [unwired: 2 in]
      n184 = Decimal String To Number(string=w459) -> (number=w456:i32)  [unwired: 2 in, 1 out]
      n185 = Decimal String To Number(string=w458) -> (number=w457:i32)  [unwired: 2 in, 1 out]
      n186 = Decimal String To Number(string=w449) -> (number=w452:i32)  [unwired: 2 in, 1 out]
      n187 = Decimal String To Number(string=w440) -> (number=w442:i32)  [unwired: 2 in, 1 out]
      n188 = Decimal String To Number(string=w450) -> (number=w451:i32)  [unwired: 2 in, 1 out]
      n189 = Decimal String To Number(string=w444) -> (number=w443:i32)  [unwired: 2 in, 1 out]
      n190 = Decimal String To Number(string=w433) -> (number=w432:i32)  [unwired: 2 in, 1 out]
      n191 = Decimal String To Number(string=w430) -> (number=w431:i32)  [unwired: 2 in, 1 out]
      n192 = Equal?(x=w464, y=w463) -> (x = y?=w462:bool)
      n193 = Subtract(x=w457, y=w456) -> (x-y=w461:i32)
      n194 = Subtract(x=w451, y=w452) -> (x-y=w448:i32)
      n195 = Subtract(x=w443, y=w442) -> (x-y=w445:i32)
      n196 = Subtract(x=w431, y=w432) -> (x-y=w429:i32)
      n197 = Increment(x=w461) -> (x+1=w455:i32)
      n198 = Increment(x=w448) -> (x+1=w453:i32)
      n199 = Increment(x=w445) -> (x+1=w441:i32)
      n200 = Increment(x=w429) -> (x+1=w422:i32)
      n201 = String Subset(string=w427, offset (0)=w432, length (rest)=w422) -> (substring=w416:string)
      n202 = String Subset(string=w427, offset (0)=w456, length (rest)=w455) -> (substring=w454:string)
      n203 = String Subset(string=w427, offset (0)=w452, length (rest)=w453) -> (substring=w446:string)
      n204 = String Subset(string=w427, offset (0)=w442, length (rest)=w441) -> (substring=w435:string)
      n205 = Decimal String To Number(string=w416) -> (number=w423:i32)  [unwired: 2 in, 1 out]
      n206 = case shown="真" w462 {
        tunnel: w454 -> [w480 w496]
        tunnel: w446 -> [w479 w494]
        tunnel: w435 -> [w477 w495]
        tunnel: w416 -> [w471 w483]
        tunnel: [w470 w484] -> w424
        frame False {
          w478 = "/"
          # "年的起始位和结束位不一样一样，则日期类型为年年月月日日"
          # "2位天数"
          # "2位月份"
          # "2位年份"
          n207 = Format Date/Time String(time format string (%c)="%H:%M:%S" ("时间格式字符串(%c)")) -> (date/time string=w475:string)  [unwired: 2 in]
          n208 = Concatenate Strings(w475, "20", w480, w478, w479, w478, w477) -> (w474:string)
          n209 = property on="show_date" class="AbsTime (严格)"("NumText.Text"=w474) -> ("Value"=w470:timestamp)  [unwired: 2 in, 2 out]
          n210 = local write "show_date"(w470) -> ()
          n211 = Format Date/Time String(time format string (%c)="%y%j" ("时间格式字符串(%c)"), seconds (now)=w470) -> (date/time string=w473:string)  [unwired: 1 in]
          n212 = Concatenate Strings(w473, w471) -> (w469:string)
          n213 = local write "show_str_yydddxxxx"(w469) -> ()
        }
        frame True {
          w489 = "/"
          # "NO W X Y Z"
          # "年的起始位和结束位一样，则日期类型为年月日"
          n214 = case shown="\"6\"" w496 {
            tunnel: [_ "2015" "2016"] -> w493
            frame Default {
            }
            frame "5" {
            }
            frame "6" {
            }
          }
          n215 = case shown="\"C\"" w494 {
            tunnel: [_ "01" "02" "03" "04" "05" "06" "07" "08" "09" "10" "11" "12"] -> w490
            frame "", Default {
            }
            frame "1" {
            }
            frame "2" {
            }
            frame "3" {
            }
            frame "4" {
            }
            frame "5" {
            }
            frame "6" {
            }
            frame "7" {
            }
            frame "8" {
            }
            frame "9" {
            }
            frame "A" {
            }
            frame "B" {
            }
            frame "C" {
            }
          }
          n216 = case shown="\"V\"" w495 {
            tunnel: [_ "01" "02" "03" "04" "05" "06" "07" "08" "09" "10" "11" "12" "13" "14" "15" "16" "17" "18" "19" "20" "21" "22" "23" "24" "25" "26" "27" "28" "29" "30" "31"] -> w488
            frame "", Default {
            }
            frame "1" {
            }
            frame "2" {
            }
            frame "3" {
            }
            frame "4" {
            }
            frame "5" {
            }
            frame "6" {
            }
            frame "7" {
            }
            frame "8" {
            }
            frame "9" {
            }
            frame "A" {
            }
            frame "B" {
            }
            frame "C" {
            }
            frame "D" {
            }
            frame "E" {
            }
            frame "F" {
            }
            frame "G" {
            }
            frame "H" {
            }
            frame "I" {
            }
            frame "J" {
            }
            frame "K" {
            }
            frame "L" {
            }
            frame "M" {
            }
            frame "N" {
            }
            frame "O" {
            }
            frame "P" {
            }
            frame "Q" {
            }
            frame "R" {
            }
            frame "S" {
            }
            frame "T" {
            }
            frame "U" {
            }
            frame "V" {
            }
          }
          n217 = Format Date/Time String(time format string (%c)="%H:%M:%S" ("时间格式字符串(%c)")) -> (date/time string=w491:string)  [unwired: 2 in]
          n218 = Concatenate Strings(w491, w493, w489, w490, w489, w488) -> (w487:string)
          n219 = property on="show_date" class="AbsTime (严格)"("NumText.Text"=w487) -> ("Value"=w484:timestamp)  [unwired: 2 in, 2 out]
          n220 = local write "show_date"(w484) -> ()
          n221 = Format Date/Time String(time format string (%c)="%y%j" ("时间格式字符串(%c)"), seconds (now)=w484) -> (date/time string=w485:string)  [unwired: 1 in]
          n222 = Concatenate Strings(w485, w483) -> (w482:string)
          n223 = local write "show_str_yydddxxxx"(w482) -> ()
        }
      }
      n224 = local write "show_int_Xn"(w423) -> ()
      n225 = call "36StrToDecStr_dell.vi"("input_str_hex"=w416) -> ("数值"=w415:i32)
      n226 = Number To Decimal String(number=w415, width (-)=w422) -> (decimal integer string=w421:string)
      n227 = Search and Replace String(replace all?=TRUE ("替换全部？(F)"), input string=w421, search string=" " ("搜索字符串"), replace string="0" ("替换字符串(\"\")")) -> (result string=w417:string)  [unwired: 4 in, 3 out]
      n228 = disable-structure shown="禁用" {
        frame Disabled {
          n229 = call "25StrToDecStr_dell.vi"() -> ()  [unwired: 1 in, 1 out]
        }
        frame Enabled {
        }
      }
    }
    frame "NoDate" {
      # "结束位"
      # "起始位"
      n230 = Array Subset(array=w546, index=9 ("索引"), length=2 ("长度")) -> (w548:string[])
      n231 = Index Array(array=w548, index #1=0 ("索引")) -> (element #1=w553:string, element #2=w550:string)  [unwired: 1 in]
      n232 = Decimal String To Number(string=w553) -> (number=w552:i32)  [unwired: 2 in, 1 out]
      n233 = Decimal String To Number(string=w550) -> (number=w551:i32)  [unwired: 2 in, 1 out]
      n234 = Subtract(x=w551, y=w552) -> (x-y=w549:i32)
      n235 = Increment(x=w549) -> (x+1=w547:i32)
      n236 = String Subset(string=w543, offset (0)=w552, length (rest)=w547) -> (substring=w544:string)
      n237 = Get Date/Time In Seconds() -> (seconds since 1Jan1904=w542:timestamp)
    }
    frame "年月日3" {
      w560 = 2 ("索引")
      # "结束位"
      # "起始位"
      # "结束位"
      # "起始位"
      # "结束位"
      # "起始位"
      # "结束位"
      # "起始位"
      # "日期类型为“年月日”，则需读取配置中的1、2、3、4、7、8、9、10"
      n238 = local read "input_str_label"() -> (w562:string)
      n239 = Array Subset(array=w600, index=1 ("索引"), length=w560) -> (w595:string[])
      n240 = Array Subset(array=w600, index=3 ("索引"), length=w560) -> (w582:string[])
      n241 = Array Subset(array=w600, index=7 ("索引"), length=w560) -> (w574:string[])
      n242 = Array Subset(array=w600, index=9 ("索引"), length=w560) -> (w563:string[])
      n243 = Index Array(array=w595, index #1=0 ("索引")) -> (element #1=w594:string, element #2=w593:string)  [unwired: 1 in]
      n244 = Index Array(array=w582, index #1=0 ("索引")) -> (element #1=w584:string, element #2=w585:string)  [unwired: 1 in]
      n245 = Index Array(array=w574, index #1=0 ("索引")) -> (element #1=w575:string, element #2=w579:string)  [unwired: 1 in]
      n246 = Index Array(array=w563, index #1=0 ("索引")) -> (element #1=w568:string, element #2=w565:string)  [unwired: 1 in]
      n247 = Index Array(array=w595) -> (element #1=w599:string, element #2=w598:string)  [unwired: 2 in]
      n248 = Decimal String To Number(string=w594) -> (number=w591:i32)  [unwired: 2 in, 1 out]
      n249 = Decimal String To Number(string=w593) -> (number=w592:i32)  [unwired: 2 in, 1 out]
      n250 = Decimal String To Number(string=w584) -> (number=w587:i32)  [unwired: 2 in, 1 out]
      n251 = Decimal String To Number(string=w575) -> (number=w577:i32)  [unwired: 2 in, 1 out]
      n252 = Decimal String To Number(string=w585) -> (number=w586:i32)  [unwired: 2 in, 1 out]
      n253 = Decimal String To Number(string=w579) -> (number=w578:i32)  [unwired: 2 in, 1 out]
      n254 = Decimal String To Number(string=w568) -> (number=w567:i32)  [unwired: 2 in, 1 out]
      n255 = Decimal String To Number(string=w565) -> (number=w566:i32)  [unwired: 2 in, 1 out]
      n256 = Equal?(x=w599, y=w598) -> (x = y?=w597:bool)
      n257 = Subtract(x=w592, y=w591) -> (x-y=w596:i32)
      n258 = Subtract(x=w586, y=w587) -> (x-y=w583:i32)
      n259 = Subtract(x=w578, y=w577) -> (x-y=w580:i32)
      n260 = Subtract(x=w566, y=w567) -> (x-y=w564:i32)
      n261 = Increment(x=w596) -> (x+1=w590:i32)
      n262 = Increment(x=w583) -> (x+1=w588:i32)
      n263 = Increment(x=w580) -> (x+1=w576:i32)
      n264 = Increment(x=w564) -> (x+1=w557:i32)
      n265 = String Subset(string=w562, offset (0)=w567, length (rest)=w557) -> (substring=w556:string)
      n266 = String Subset(string=w562, offset (0)=w591, length (rest)=w590) -> (substring=w589:string)
      n267 = String Subset(string=w562, offset (0)=w587, length (rest)=w588) -> (substring=w581:string)
      n268 = String Subset(string=w562, offset (0)=w577, length (rest)=w576) -> (substring=w570:string)
      n269 = Decimal String To Number(string=w556) -> (number=w558:i32)  [unwired: 2 in, 1 out]
      n270 = case shown="真" w597 {
        tunnel: w589 -> [w622 w638]
        tunnel: w581 -> [w621 w636]
        tunnel: w570 -> [w619 w637]
        tunnel: w556 -> [w613 w625]
        tunnel: [w612 w626] -> w559
        frame False {
          w620 = "/"
          # "年的起始位和结束位不一样一样，则日期类型为年年月月日日"
          # "2位天数"
          # "2位月份"
          # "2位年份"
          n271 = Format Date/Time String(time format string (%c)="%H:%M:%S" ("时间格式字符串(%c)")) -> (date/time string=w617:string)  [unwired: 2 in]
          n272 = Concatenate Strings(w617, "20", w622, w620, w621, w620, w619) -> (w616:string)
          n273 = property on="show_date" class="AbsTime (严格)"("NumText.Text"=w616) -> ("Value"=w612:timestamp)  [unwired: 2 in, 2 out]
          n274 = local write "show_date"(w612) -> ()
          n275 = Format Date/Time String(time format string (%c)="%y%j" ("时间格式字符串(%c)"), seconds (now)=w612) -> (date/time string=w615:string)  [unwired: 1 in]
          n276 = Concatenate Strings(w615, w613) -> (w611:string)
          n277 = local write "show_str_yydddxxxx"(w611) -> ()
        }
        frame True {
          w631 = "/"
          # "WXYZ"
          # "年的起始位和结束位一样，则日期类型为年月日"
          n278 = case shown="\"6\"" w638 {
            tunnel: [_ "2015" "2016"] -> w635
            frame Default {
            }
            frame "5" {
            }
            frame "6" {
            }
          }
          n279 = case shown="\"C\"" w636 {
            tunnel: [_ "01" "02" "03" "04" "05" "06" "07" "08" "09" "10" "11" "12"] -> w632
            frame "", Default {
            }
            frame "1" {
            }
            frame "2" {
            }
            frame "3" {
            }
            frame "4" {
            }
            frame "5" {
            }
            frame "6" {
            }
            frame "7" {
            }
            frame "8" {
            }
            frame "9" {
            }
            frame "A" {
            }
            frame "B" {
            }
            frame "C" {
            }
          }
          n280 = case shown="\"V\"" w637 {
            tunnel: [_ "01" "02" "03" "04" "05" "06" "07" "08" "09" "10" "11" "12" "13" "14" "15" "16" "17" "18" "19" "20" "21" "22" "23" "24" "25" "26" "27" "28" "29" "30" "31"] -> w630
            frame "", Default {
            }
            frame "1" {
            }
            frame "2" {
            }
            frame "3" {
            }
            frame "4" {
            }
            frame "5" {
            }
            frame "6" {
            }
            frame "7" {
            }
            frame "8" {
            }
            frame "9" {
            }
            frame "A" {
            }
            frame "B" {
            }
            frame "C" {
            }
            frame "D" {
            }
            frame "E" {
            }
            frame "F" {
            }
            frame "G" {
            }
            frame "H" {
            }
            frame "I" {
            }
            frame "J" {
            }
            frame "K" {
            }
            frame "L" {
            }
            frame "M" {
            }
            frame "N" {
            }
            frame "O" {
            }
            frame "P" {
            }
            frame "Q" {
            }
            frame "R" {
            }
            frame "S" {
            }
            frame "T" {
            }
            frame "U" {
            }
            frame "V" {
            }
          }
          n281 = Format Date/Time String(time format string (%c)="%H:%M:%S" ("时间格式字符串(%c)")) -> (date/time string=w633:string)  [unwired: 2 in]
          n282 = Concatenate Strings(w633, w635, w631, w632, w631, w630) -> (w629:string)
          n283 = property on="show_date" class="AbsTime (严格)"("NumText.Text"=w629) -> ("Value"=w626:timestamp)  [unwired: 2 in, 2 out]
          n284 = local write "show_date"(w626) -> ()
          n285 = Format Date/Time String(time format string (%c)="%y%j" ("时间格式字符串(%c)"), seconds (now)=w626) -> (date/time string=w627:string)  [unwired: 1 in]
          n286 = Concatenate Strings(w627, w625) -> (w624:string)
          n287 = local write "show_str_yydddxxxx"(w624) -> ()
        }
      }
      n288 = local write "show_int_Xn"(w558) -> ()
      n289 = disable-structure shown="禁用" {
        disable-tunnel: w557 -> [w609 _]
        disable-tunnel: [w604 _] -> _
        frame Disabled {
          n290 = call "25StrToDecStr_dell.vi"() -> ("数值"=w610:i32)  [unwired: 1 in]
          n291 = Number To Decimal String(number=w610, width (-)=w609) -> (decimal integer string=w608:string)
          n292 = Search and Replace String(replace all?=TRUE ("替换全部？(F)"), input string=w608, search string=" " ("搜索字符串"), replace string="0" ("替换字符串(\"\")")) -> (result string=w604:string)  [unwired: 4 in, 3 out]
        }
        frame Enabled {
        }
      }
    }
    frame "年周" {
      w698 = 2 ("索引")
      w730 = "/"
      # "得到本周一在本月的天数"
      # "减去首尾周的天数"
      # "如何由周数+本周一计算出本月天数？\n由周数-2，加本周周一，计算出天数，\n然后减去上个月的天数"
      # "如何由周数计算出月份？\n由周数-2，加本周周一，计算出天数\n再根据12月份的天数范围去匹配"
      # "日期类型为“年周”实际是“年年周周”，天数按照当天去补"
      # "2位天数"
      # "2位周数"
      # "2位年份"
      # "日期类型为“年周”，则需读取配置中的1、2、5、6、9、10"
      # "结束位"
      # "起始位"
      # "结束位"
      # "起始位"
      # "结束位"
      # "起始位"
      n293 = local read "input_str_label"() -> (w732:string)
      n294 = Array Subset(array=w756, index=1 ("索引"), length=w698) -> (w726:string[])
      n295 = Array Subset(array=w756, index=5 ("索引"), length=w698) -> (w743:string[])
      n296 = Array Subset(array=w756, index=9 ("索引"), length=w698) -> (w733:string[])
      n297 = Index Array(array=w726, index #1=0 ("索引")) -> (element #1=w754:string, element #2=w753:string)  [unwired: 1 in]
      n298 = Index Array(array=w743, index #1=0 ("索引")) -> (element #1=w745:string, element #2=w746:string)  [unwired: 1 in]
      n299 = Index Array(array=w733, index #1=0 ("索引")) -> (element #1=w739:string, element #2=w735:string)  [unwired: 1 in]
      n300 = Decimal String To Number(string=w754) -> (number=w751:i32)  [unwired: 2 in, 1 out]
      n301 = Decimal String To Number(string=w753) -> (number=w752:i32)  [unwired: 2 in, 1 out]
      n302 = Decimal String To Number(string=w745) -> (number=w748:i32)  [unwired: 2 in, 1 out]
      n303 = Decimal String To Number(string=w746) -> (number=w747:i32)  [unwired: 2 in, 1 out]
      n304 = Decimal String To Number(string=w739) -> (number=w737:i32)  [unwired: 2 in, 1 out]
      n305 = Decimal String To Number(string=w735) -> (number=w736:i32)  [unwired: 2 in, 1 out]
      n306 = Subtract(x=w752, y=w751) -> (x-y=w755:i32)
      n307 = Subtract(x=w747, y=w748) -> (x-y=w744:i32)
      n308 = Subtract(x=w736, y=w737) -> (x-y=w734:i32)
      n309 = Increment(x=w755) -> (x+1=w750:i32)
      n310 = Increment(x=w744) -> (x+1=w749:i32)
      n311 = Increment(x=w734) -> (x+1=w738:i32)
      n312 = String Subset(string=w732, offset (0)=w737, length (rest)=w738) -> (substring=w699:string)
      n313 = String Subset(string=w732, offset (0)=w751, length (rest)=w750) -> (substring=w691:string)
      n314 = String Subset(string=w732, offset (0)=w748, length (rest)=w749) -> (substring=w725:string)
      n315 = Search and Replace String(input string="20:15:00\n20Y/01/01" ("时间格式字符串(%c)"), search string="Y" ("搜索字符串"), replace string=w691) -> (result string=w694:string)  [unwired: 5 in, 3 out]
      n316 = Decimal String To Number(string=w725) -> (number=w689:i32)  [unwired: 2 in, 1 out]
      n317 = Format Date/Time String(time format string (%c)=w694) -> (date/time string=w724:string)  [unwired: 2 in]
      n318 = Decimal String To Number(string=w699) -> (number=w703:i32)  [unwired: 2 in, 1 out]
      n319 = property on="midVar_date_1" class="AbsTime (严格)"("NumText.Text"=w724) -> ("Value"=w723:timestamp)  [unwired: 2 in, 2 out]
      n320 = local write "show_int_Xn"(w703) -> ()
      n321 = Format Date/Time String(time format string (%c)="%w" ("时间格式字符串(%c)"), seconds (now)=w723) -> (date/time string=w720:string)  [unwired: 1 in]
      n322 = Decimal String To Number(string=w720) -> (number=w719:i32)  [unwired: 2 in, 1 out]
      n323 = Subtract(x=7, y=w719) -> (x-y=w718:i32)
      n324 = Increment(x=w718) -> (x+1=w688:i32)
      n325 = Search and Replace String(input string="20Y/" ("时间格式字符串(%c)"), search string="Y" ("搜索字符串"), replace string=w691) -> (result string=w690:string)  [unwired: 5 in, 3 out]
      n326 = call "dealWithWeek.vi"("input_day"=1, "input_firstWeek"=w688, "input_week"=w689) -> ("ddd"=w687:i32)  [unwired: 8 in]
      n327 = Format Date/Time String(time format string (%c)=w690) -> (date/time string=w716:string)  [unwired: 2 in]
      n328 = case shown="32..59" w687 {
        tunnel: ["01" "02" "03" "04" "05" "06" "07" "08" "09" "10" "11" "12"] -> w701
        frame 1..31, Default {
        }
        frame 32..59 {
        }
        frame 60..90 {
        }
        frame 91..120 {
        }
        frame 121..151 {
        }
        frame 152..181 {
        }
        frame 182..212 {
        }
        frame 213..243 {
        }
        frame 244..273 {
        }
        frame 274..304 {
        }
        frame 305..334 {
        }
        frame 335..365 {
        }
      }
      n329 = Format Date/Time String(time format string (%c)="%H:%M:%S" ("时间格式字符串(%c)")) -> (date/time string=w713:string)  [unwired: 2 in]
      n330 = Concatenate Strings(w713, w716, w701, "/01") -> (w714:string)
      n331 = property on="midVar_date_2" class="AbsTime (严格)"("NumText.Text"=w714) -> ("Value"=w712:timestamp)  [unwired: 2 in, 2 out]
      n332 = Format Date/Time String(time format string (%c)="%j" ("时间格式字符串(%c)"), seconds (now)=w712) -> (date/time string=w710:string)  [unwired: 1 in]
      n333 = Decimal String To Number(string=w710) -> (number=w709:i32)  [unwired: 2 in, 1 out]
      n334 = Decrement(x=w709) -> (x-1=w700:i32)
      n335 = Format Date/Time String(time format string (%c)="%H:%M:%S" ("时间格式字符串(%c)")) -> (date/time string=w728:string)  [unwired: 2 in]
      n336 = Subtract(x=w687, y=w700) -> (x-y=w708:i32)
      n337 = call "intToNWidthString.vi"("input_int_width"=2, "input_int_number"=w708) -> ("show_str_number"=w707:string)
      n338 = Concatenate Strings(w728, "20", w691, w730, w701, w730, w707) -> (w727:string)
      n339 = property on="show_date" class="AbsTime (严格)"("NumText.Text"=w727) -> ("Value"=w684:timestamp)  [unwired: 2 in, 2 out]
      n340 = Format Date/Time String(time format string (%c)="%y%j" ("时间格式字符串(%c)"), seconds (now)=w684) -> (date/time string=w705:string)  [unwired: 1 in]
      n341 = Concatenate Strings(w705, w699) -> (w704:string)
      n342 = local write "show_str_yydddxxxx"(w704) -> ()
      n343 = local write "show_date"(w684) -> ()
      n344 = Get Date/Time In Seconds() -> (seconds since 1Jan1904=w685:timestamp)
      n345 = Subtract(x=w685, y=w684) -> ()  [unwired: 1 out]
    }
    frame "年周天" {
      w780 = 2 ("索引")
      w830 = "/"
      # "如何计算之前月份的所有天数？\n用本月1号来算，结果减去1即可"
      # "结束位"
      # "起始位"
      # "得到本周一在本月的天数"
      # "减去首尾周的天数"
      # "如何由周数+本周一计算出本月天数？\n由周数-2，加本周周一，计算出天数，\n然后减去前所有月的天数"
      # "如何由周数计算出月份？\n由周数-2，加本周周一，计算出天数\n再根据12月份的天数范围去匹配"
      # "日期类型为“年周天”实际是“年年周周天”"
      # "2位天数"
      # "2位周数"
      # "2位年份"
      # "日期类型为“年周天”，则需读取配置中的1、2、5、6、7、8、9、10"
      # "结束位"
      # "起始位"
      # "结束位"
      # "起始位"
      # "结束位"
      # "起始位"
      n346 = local read "input_str_label"() -> (w791:string)
      n347 = Array Subset(array=w792, index=7 ("索引"), length=w780) -> (w800:string[])
      n348 = Array Subset(array=w792, index=1 ("索引"), length=w780) -> (w827:string[])
      n349 = Array Subset(array=w792, index=5 ("索引"), length=w780) -> (w842:string[])
      n350 = Array Subset(array=w792, index=9 ("索引"), length=w780) -> (w832:string[])
      n351 = Index Array(array=w827, index #1=0 ("索引")) -> (element #1=w853:string, element #2=w852:string)  [unwired: 1 in]
      n352 = Index Array(array=w800, index #1=0 ("索引")) -> (element #1=w798:string, element #2=w797:string)  [unwired: 1 in]
      n353 = Index Array(array=w842, index #1=0 ("索引")) -> (element #1=w844:string, element #2=w845:string)  [unwired: 1 in]
      n354 = Index Array(array=w832, index #1=0 ("索引")) -> (element #1=w838:string, element #2=w834:string)  [unwired: 1 in]
      n355 = Decimal String To Number(string=w853) -> (number=w850:i32)  [unwired: 2 in, 1 out]
      n356 = Decimal String To Number(string=w852) -> (number=w851:i32)  [unwired: 2 in, 1 out]
      n357 = Decimal String To Number(string=w798) -> (number=w795:i32)  [unwired: 2 in, 1 out]
      n358 = Decimal String To Number(string=w844) -> (number=w847:i32)  [unwired: 2 in, 1 out]
      n359 = Decimal String To Number(string=w797) -> (number=w796:i32)  [unwired: 2 in, 1 out]
      n360 = Decimal String To Number(string=w845) -> (number=w846:i32)  [unwired: 2 in, 1 out]
      n361 = Decimal String To Number(string=w838) -> (number=w836:i32)  [unwired: 2 in, 1 out]
      n362 = Decimal String To Number(string=w834) -> (number=w835:i32)  [unwired: 2 in, 1 out]
      n363 = Subtract(x=w851, y=w850) -> (x-y=w854:i32)
      n364 = Subtract(x=w796, y=w795) -> (x-y=w799:i32)
      n365 = Subtract(x=w846, y=w847) -> (x-y=w843:i32)
      n366 = Subtract(x=w835, y=w836) -> (x-y=w833:i32)
      n367 = Increment(x=w854) -> (x+1=w849:i32)
      n368 = Increment(x=w799) -> (x+1=w794:i32)
      n369 = Increment(x=w843) -> (x+1=w848:i32)
      n370 = Increment(x=w833) -> (x+1=w837:i32)
      n371 = String Subset(string=w791, offset (0)=w836, length (rest)=w837) -> (substring=w778:string)
      n372 = String Subset(string=w791, offset (0)=w795, length (rest)=w794) -> (substring=w783:string)
      n373 = String Subset(string=w791, offset (0)=w850, length (rest)=w849) -> (substring=w786:string)
      n374 = String Subset(string=w791, offset (0)=w847, length (rest)=w848) -> (substring=w785:string)
      n375 = Decimal String To Number(string=w783) -> (number=w775:i32)  [unwired: 2 in, 1 out]
      n376 = Format Date/Time String(time format string (%c)="20:15:00\n%Y/01/01" ("时间格式字符串(%c)")) -> (date/time string=w824:string)  [unwired: 2 in]
      n377 = Decimal String To Number(string=w785) -> (number=w774:i32)  [unwired: 2 in, 1 out]
      n378 = Concatenate Strings(w786, w785, "S", w783) -> (→"show_str_yywwSd":string)
      n379 = Decimal String To Number(string=w778) -> (number=w803:i32)  [unwired: 2 in, 1 out]
      n380 = property on="midVar_date_1" class="AbsTime (严格)"("NumText.Text"=w824) -> ("Value"=w823:timestamp)  [unwired: 2 in, 2 out]
      n381 = Equal To 0?(x=w775) -> (x = 0?=w777:bool)
      n382 = local write "show_int_Xn"(w803) -> ()
      n383 = Select(t=7, s=w777, f=w775) -> (s? t:f=w772:i32)
      n384 = Format Date/Time String(time format string (%c)="%w" ("时间格式字符串(%c)"), seconds (now)=w823) -> (date/time string=w820:string)  [unwired: 1 in]
      n385 = Decimal String To Number(string=w820) -> (number=w819:i32)  [unwired: 2 in, 1 out]
      n386 = Subtract(x=7, y=w819) -> (x-y=w818:i32)
      n387 = Increment(x=w818) -> (x+1=w773:i32)
      n388 = call "dealWithWeek.vi"("input_day"=w772, "input_firstWeek"=w773, "input_week"=w774) -> ("ddd"=w771:i32)  [unwired: 8 in]
      n389 = Format Date/Time String(time format string (%c)="%Y/" ("时间格式字符串(%c)")) -> (date/time string=w816:string)  [unwired: 2 in]
      n390 = Format Date/Time String(time format string (%c)="%H:%M:%S" ("时间格式字符串(%c)")) -> (date/time string=w813:string)  [unwired: 2 in]
      n391 = case shown="335..365" w771 {
        tunnel: ["01" "02" "03" "04" "05" "06" "07" "08" "09" "10" "11" "12"] -> w790
        frame 1..31, Default {
        }
        frame 32..59 {
        }
        frame 60..90 {
        }
        frame 91..120 {
        }
        frame 121..151 {
        }
        frame 152..181 {
        }
        frame 182..212 {
        }
        frame 213..243 {
        }
        frame 244..273 {
        }
        frame 274..304 {
        }
        frame 305..334 {
        }
        frame 335..365 {
        }
      }
      n392 = Concatenate Strings(w813, w816, w790, "/01") -> (w814:string)
      n393 = property on="midVar_date_2" class="AbsTime (严格)"("NumText.Text"=w814) -> ("Value"=w812:timestamp)  [unwired: 2 in, 2 out]
      n394 = Format Date/Time String(time format string (%c)="%j" ("时间格式字符串(%c)"), seconds (now)=w812) -> (date/time string=w810:string)  [unwired: 1 in]
      n395 = Decimal String To Number(string=w810) -> (number=w809:i32)  [unwired: 2 in, 1 out]
      n396 = Format Date/Time String(time format string (%c)="%H:%M:%S" ("时间格式字符串(%c)")) -> (date/time string=w788:string)  [unwired: 2 in]
      n397 = Decrement(x=w809) -> (x-1=w789:i32)
      n398 = Subtract(x=w771, y=w789) -> (x-y=w808:i32)
      n399 = call "intToNWidthString.vi"("input_int_width"=2, "input_int_number"=w808) -> ("show_str_number"=w807:string)
      n400 = Concatenate Strings(w788, "\n", "20", w786, w830, w790, w830, w807) -> (w828:string)
      n401 = property on="show_date" class="AbsTime (严格)"("NumText.Text"=w828) -> ("Value"=w779:timestamp)  [unwired: 2 in, 2 out]
      n402 = Format Date/Time String(time format string (%c)="%y%j" ("时间格式字符串(%c)"), seconds (now)=w779) -> (date/time string=w805:string)  [unwired: 1 in]
      n403 = Concatenate Strings(w805, w778) -> (w804:string)
      n404 = local write "show_str_yydddxxxx"(w804) -> ()
      n405 = local write "show_date"(w779) -> ()
    }
    frame "年天" {
      w881 = 2 ("索引")
      w904 = "/"
      # "计算出月份"
      # "天数"
      # "输出月份"
      # "天"
      # "结束位"
      # "起始位"
      # "如何计算之前月份的所有天数？\n用本月1号来算，结果减去1即可"
      # "日期类型为“年天”实际是“年年天天天”"
      # "2位年份"
      # "日期类型为“年周天”，则需读取配置中的1、2、9、10"
      # "结束位"
      # "起始位"
      # "结束位"
      # "起始位"
      n406 = local read "input_str_label"() -> (w896:string)
      n407 = Array Subset(array=w882, index=7 ("索引"), length=w881) -> (w889:string[])
      n408 = Array Subset(array=w882, index=1 ("索引"), length=w881) -> (w901:string[])
      n409 = Array Subset(array=w882, index=9 ("索引"), length=w881) -> (w906:string[])
      n410 = Index Array(array=w889, index #1=0 ("索引")) -> (element #1=w885:string, element #2=w887:string)  [unwired: 1 in]
      n411 = Index Array(array=w901, index #1=0 ("索引")) -> (element #1=w919:string, element #2=w918:string)  [unwired: 1 in]
      n412 = Index Array(array=w906, index #1=0 ("索引")) -> (element #1=w912:string, element #2=w908:string)  [unwired: 1 in]
      n413 = Decimal String To Number(string=w885) -> (number=w879:i32)  [unwired: 2 in, 1 out]
      n414 = Decimal String To Number(string=w887) -> (number=w886:i32)  [unwired: 2 in, 1 out]
      n415 = Decimal String To Number(string=w919) -> (number=w916:i32)  [unwired: 2 in, 1 out]
      n416 = Decimal String To Number(string=w918) -> (number=w917:i32)  [unwired: 2 in, 1 out]
      n417 = Decimal String To Number(string=w912) -> (number=w910:i32)  [unwired: 2 in, 1 out]
      n418 = Decimal String To Number(string=w908) -> (number=w909:i32)  [unwired: 2 in, 1 out]
      n419 = Subtract(x=w886, y=w879) -> (x-y=w888:i32)
      n420 = Subtract(x=w917, y=w916) -> (x-y=w920:i32)
      n421 = Subtract(x=w909, y=w910) -> (x-y=w907:i32)
      n422 = Increment(x=w888) -> (x+1=w880:i32)
      n423 = Increment(x=w920) -> (x+1=w915:i32)
      n424 = Increment(x=w907) -> (x+1=w911:i32)
      n425 = String Subset(string=w896, offset (0)=w910, length (rest)=w911) -> (substring=w890:string)
      n426 = String Subset(string=w896, offset (0)=w879, length (rest)=w880) -> (substring=w878:string)
      n427 = String Subset(string=w896, offset (0)=w916, length (rest)=w915) -> (substring=w893:string)
      n428 = Decimal String To Number(string=w878) -> (number=w871:i32)  [unwired: 2 in, 1 out]
      n429 = Decimal String To Number(string=w890) -> (number=w897:i32)  [unwired: 2 in, 1 out]
      n430 = case shown="32..60" w871 {
        selector: w871 -> [w922 w925 w928 w931 w934 w937 w940 w943 w946 w949 w952 w955]
        tunnel: [w922 w923 w926 w929 w932 w935 w938 w941 w944 w947 w950 w953] -> w876
        frame 1..31, Default {
        }
        frame 32..60 {
          n431 = Subtract(x=w925, y=31) -> (x-y=w923:i32)
        }
        frame 61..91 {
          n432 = Subtract(x=w928, y=60) -> (x-y=w926:i32)
        }
        frame 92..121 {
          n433 = Subtract(x=w931, y=91) -> (x-y=w929:i32)
        }
        frame 122..152 {
          n434 = Subtract(x=w934, y=121) -> (x-y=w932:i32)
        }
        frame 153..183 {
          n435 = Subtract(x=w937, y=152) -> (x-y=w935:i32)
        }
        frame 184..213 {
          n436 = Subtract(x=w940, y=183) -> (x-y=w938:i32)
        }
        frame 214..244 {
          n437 = Subtract(x=w943, y=213) -> (x-y=w941:i32)
        }
        frame 245..274 {
          n438 = Subtract(x=w946, y=244) -> (x-y=w944:i32)
        }
        frame 275..305 {
          n439 = Subtract(x=w949, y=275) -> (x-y=w947:i32)
        }
        frame 306..335 {
          n440 = Subtract(x=w952, y=305) -> (x-y=w950:i32)
        }
        frame 336..366 {
          n441 = Subtract(x=w955, y=335) -> (x-y=w953:i32)
        }
      }
      n442 = case shown="61..91" w871 {
        tunnel: ["01" "02" "03" "04" "05" "06" "07" "08" "09" "10" "11" "12"] -> _
        frame 1..31, Default {
        }
        frame 32..60 {
        }
        frame 61..91 {
        }
        frame 92..121 {
        }
        frame 122..152 {
        }
        frame 153..183 {
        }
        frame 184..213 {
        }
        frame 214..244 {
        }
        frame 245..274 {
        }
        frame 275..305 {
        }
        frame 306..335 {
        }
        frame 336..366 {
        }
      }
      n443 = local write "show_int_Xn"(w897) -> ()
      n444 = Number To Decimal String(number=w876, width (-)=i16 2 ("宽度(-)")) -> (decimal integer string=w875:string)
      n445 = Search and Replace String(replace all?=TRUE ("替换全部？(F)"), input string=w875, search string=" " ("搜索字符串"), replace string="0" ("替换字符串(\"\")")) -> ()  [unwired: 4 in, 4 out]
      n446 = call "天数计算.vi"("天数"=w871) -> ("月份"=w869:string, "日期"=w870:string)  [unwired: 7 in, 1 out]
      n447 = Format Date/Time String(time format string (%c)="%H:%M:%S" ("时间格式字符串(%c)")) -> (date/time string=w895:string)  [unwired: 2 in]
      n448 = Concatenate Strings(w895, "\n", "20", w893, w904, w869, w904, w870) -> (w902:string)
      n449 = property on="show_date" class="AbsTime (严格)"("NumText.Text"=w902) -> ("Value"=w891:timestamp)  [unwired: 2 in, 2 out]
      n450 = Format Date/Time String(time format string (%c)="%y%j" ("时间格式字符串(%c)"), seconds (now)=w891) -> (date/time string=w899:string)  [unwired: 1 in]
      n451 = Concatenate Strings(w899, w890) -> (w898:string)
      n452 = local write "show_str_yydddxxxx"(w898) -> ()
      n453 = local write "show_date"(w891) -> ()
    }
  }
  n454 = local read "input_array_labelConfig"() -> (w5:string[])
  n455 = Index Array(array=w5, index=11 ("索引")) -> (element=w9:string)
  n456 = Index Array(array=w5, index=0 ("索引")) -> (element=w4:string)
  n457 = case shown="\"年周\"" w4 {
    tunnel: w3 -> [_ w969]
    tunnel: ["date" w969] -> w2
    frame "年周" {
    }
    frame "真", Default {
    }
  }
  n458 = call "dealWithSNType.vi"("SNXn"=w8, "SNType"=w9, "TimeInput"=w2) -> ("show_str_SNwithWholeFormat"=→"show_str_snObeyFormat":string)  [unwired: 1 out]
